vi "PRIME Detector Send CONFIG command.vi"(8 "error in (no error)":errorcluster, 9 "Integration Mode":T1, 10 "Offsets":u16[][](array[numeric])=[[0, 0, 0, 0, 0, 0, 0, 0, 0, 0, 0, 0, 0, 0, 0, 0, 0, 0, 0, 0, 0, 0, 0, 0, 0, 0, 0, 0, 0, 0, 0, 0]] format="%04x", 11 "connection ID":refnum<k5>) -> (0 "error out":errorcluster, 3 "connection ID out":refnum<k5>)   [LabVIEW 2021, in "PRIME Detector.lvclass"]
uses:
  PRIME Detector.lvclass
  Detector enum Detector Integration Mode.ctl
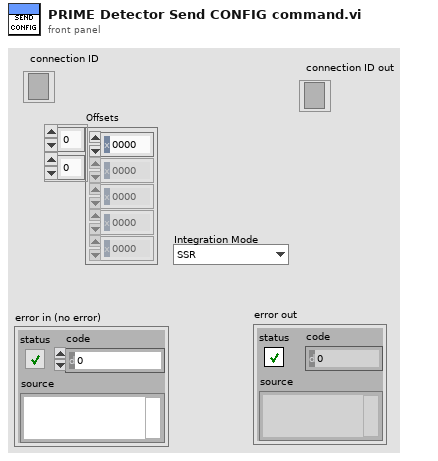
[diagram p1: front panel]
types:
  T1 = typedef "Detector enum Detector Integration Mode.ctl" = enum16{"SSR", "CDS", "MEAN", "MEDIAN", "MODE", "MIIN", "MAX"}
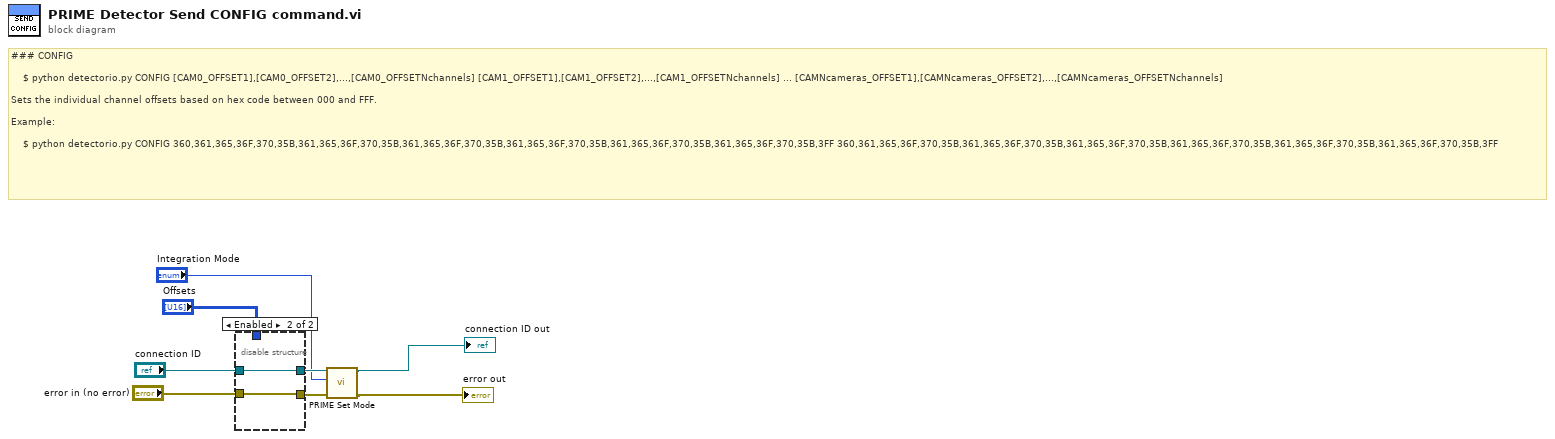
[diagram p0: block diagram]
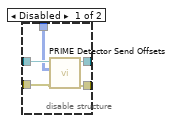
[diagram p2: hidden frame]
diagram:
  # "### CONFIG\n\n    $ python detectorio.py CONFIG [CAM0_OFFSET1],[CAM0_OFFSET2],...,[CAM0_OFFSETNchannels] [CAM1_OFFSET1],[CAM1_OFFSET2],...,[CAM1_OFFSETNchannels] ... [CAMNcameras_OFFSET1],[CAMNcameras_OFFSET2],...,[CAMNcameras_OFFSETNchannels]\n\nSets the individual channel offsets based on hex code between 000 and FFF. \n\nExample:\n\n    $ python detectorio.py CONFIG 360,361,365,36F,370,35B,361,365,36F,370,35B,361,365,36F,370,35B,361,365,36F,370,35B,361,365,36F,370,35B,361,365,36F,370,35B,3FF 360,361,365,36F,370,35B,361,365,36F,370,35B,361,365,36F,370,35B,361,365,36F,370,35B,361,365,36F,370,35B,361,365,36F,370,35B,3FF"
  n1 = disable-structure shown="Enabled" {
    disable-tunnel: "error in (no error)" -> [w13 w14]
    disable-tunnel: "connection ID" -> [w12 w15]
    disable-tunnel: "Offsets" -> [w11 _]
    disable-tunnel: [w10 w14] -> w5
    disable-tunnel: [w9 w15] -> w4
    frame Disabled {
      n2 = call "PRIME Detector Send Offsets.vi"("error in (no error)"=w13, "Offsets"=w11, "connection ID"=w12) -> ("error out"=w10:errorcluster, "connection ID out"=w9:refnum<k5>)  [unwired: 7 in]
    }
    frame Enabled {
    }
  }
  n3 = call "PRIME Set Mode.vi"("error in (no error)"=w5, "Integration Mode"="Integration Mode", "connection ID"=w4) -> ("error out"=→"error out":errorcluster, "connection ID out"=→"connection ID out":refnum<k5>)  [unwired: 6 in, 1 out]
